vi "test_Remove Speciality Input Channels.vi"(8 "error in (no error)":errorcluster, 11 "TestCase in":refnum<class "FPGA Addon Adding Channel Items Unit Tests.lvclass">) -> (0 "error out":errorcluster, 3 "TestCase out":refnum<class "FPGA Addon Adding Channel Items Unit Tests.lvclass">)   [LabVIEW 2018, in "FPGA Addon Adding Channel Items Unit Tests.lvclass"]
uses:
  FPGA Addon Adding Channel Items Unit Tests.lvclass
  Addon/Addon Shared/Types/FG Action.ctl
  FPGA Addon Adding Channel Items Unit Tests.lvclass/FPGA Addon Adding Channel Items Unit Tests.ctl
  Addon/Addon Shared/SubVIs/Constants.vi
  <vilib>/NI Veristand/Custom Device Tools/Custom Device Utility Library/NI VeriStand - Search for Item by GUID.vi
  <vilib>/NI/NI VeriStand Advanced SysDef API/SysDef API/SysDef.Property.Get.vi
  <vilib>/NI/NI VeriStand Advanced SysDef API/_SubVIs/SysDef.Property.Get.Variant.vi
  <vilib>/NI/NI VeriStand Advanced SysDef API/SysDef API/SysDef.Property.Set.vi
  <vilib>/NI/NI VeriStand Advanced SysDef API/_SubVIs/SysDef.Property.Set.Variant.vi
  <vilib>/NI/NI VeriStand Advanced SysDef API/_SubVIs/SysDef.Search.GUIDs.vi
  <vilib>/addons/_JKI Toolkits/VI Tester/TestCase.llb/TestCase.lvclass
  Addon/Addon System Explorer/FPGA Addon System Explorer.lvlib
  Addon/Addon Shared/FPGA Addon Shared.lvlib
  <vilib>/NI Veristand/Custom Device Tools/Custom Device Utility Library/Custom Device Utility Library.lvlib
  <vilib>/NI/NI VeriStand Advanced SysDef API/SysDef API/Advanced System Definition.lvlib
  C:/Program Files (x86)/National Instruments/LabVIEW 2018/vi.lib/addons/_JKI Toolkits/VI Tester/TestCase.llb/TestCase.lvclass
panel:
  out "GUIDs":string[](array[string])
  in  "remove":bool
  in  "add":bool
  out "Names":string[](array[string])
  in  "Available Registers":i32[](listbox)
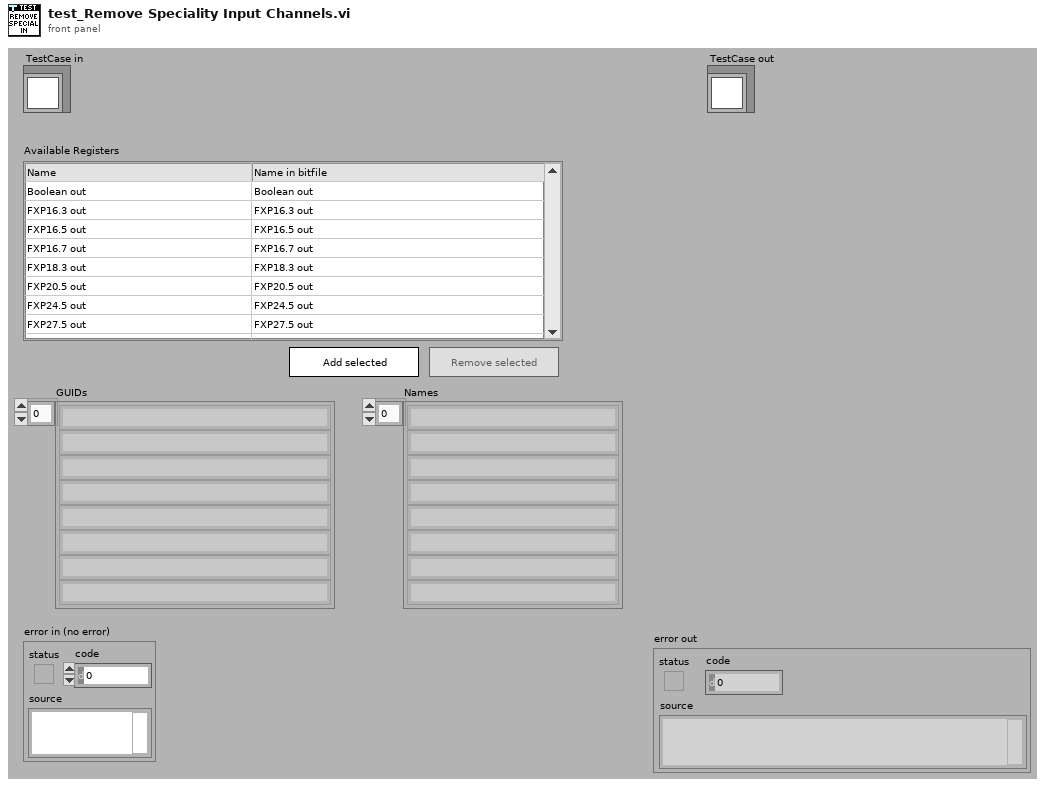
[diagram p1: front panel]
types:
  T1 = typedef "FPGA Addon Shared.lvlib/FG Action.ctl" = enum8{"GET", "SET"}
  T2 = typedef "Custom Device API.lvlib/Custom Device Item Ref.ctl" = u64
  T3 = typedef "FPGA Addon Shared.lvlib/Register Information.ctl" = cluster{"Name":string, "Data Type":T4, "Default Value":variant}
  T4 = typedef "FPGA Addon Shared.lvlib/Data Type.ctl" = enum8{"<Null>", "I8", "I16", "I32", "I64", "U8", "U16", "U32", "U64", "SGL", "Boolean", "Analog PWM In Settings", "Analog PWM In", "Digital PWM In Settings", "Digital PWM In", "Digital PWM Out", "Sine Out", "FXP+/-24.5", "FXP+/-16.5", "FXP+/-32.8", "FXP+/-64.32", "FXP+/-16.7", "FXP+/-20.5", "FXP+/-27.5", "FXP+/-32.16", "FXP+16.3", "FXP+18.3", "Digital Static In", "Digital Static Out", "Digital Static In Settings", "Digital WSS Out", "Quad Encoder Settings", "Quad Encoder In", "Group"}
  T5 = typedef "FPGA Addon System Explorer.lvlib/Listbox Cluster.ctl" = cluster{"add":refnum<vi>, "remove":refnum<vi>, "Listbox":refnum<vi>, "selected":i32[], "not present":i32[], "listbox text":string[][], "Section Ref":T2}
  T6 = typedef "Advanced System Definition.lvlib/TreeItem.Info.ctl" = cluster{"Name":string, "Description":string, "GUID":string, "Is Channel":bool, "Channel":T7, "Is Waveform":bool, "Waveform":T9}
  T7 = typedef "Custom Device API.lvlib/Custom Device Channel.ctl" = cluster{"Type":T8, "Units":string, "Default Value":dbl, "Faultable":bool, "Scalable":bool}
  T8 = typedef "Custom Device API.lvlib/Custom Device Channel Type.ctl" = enum16{"Input", "Output"}
  T9 = typedef "Custom Device API.lvlib/Custom Device Waveform.ctl" = cluster{"Data Type":T10, "Units":string}
  T10 = typedef "Custom Device API.lvlib/Custom Device Waveform DataType.ctl" = enum16{"Double", "Complex Double"}
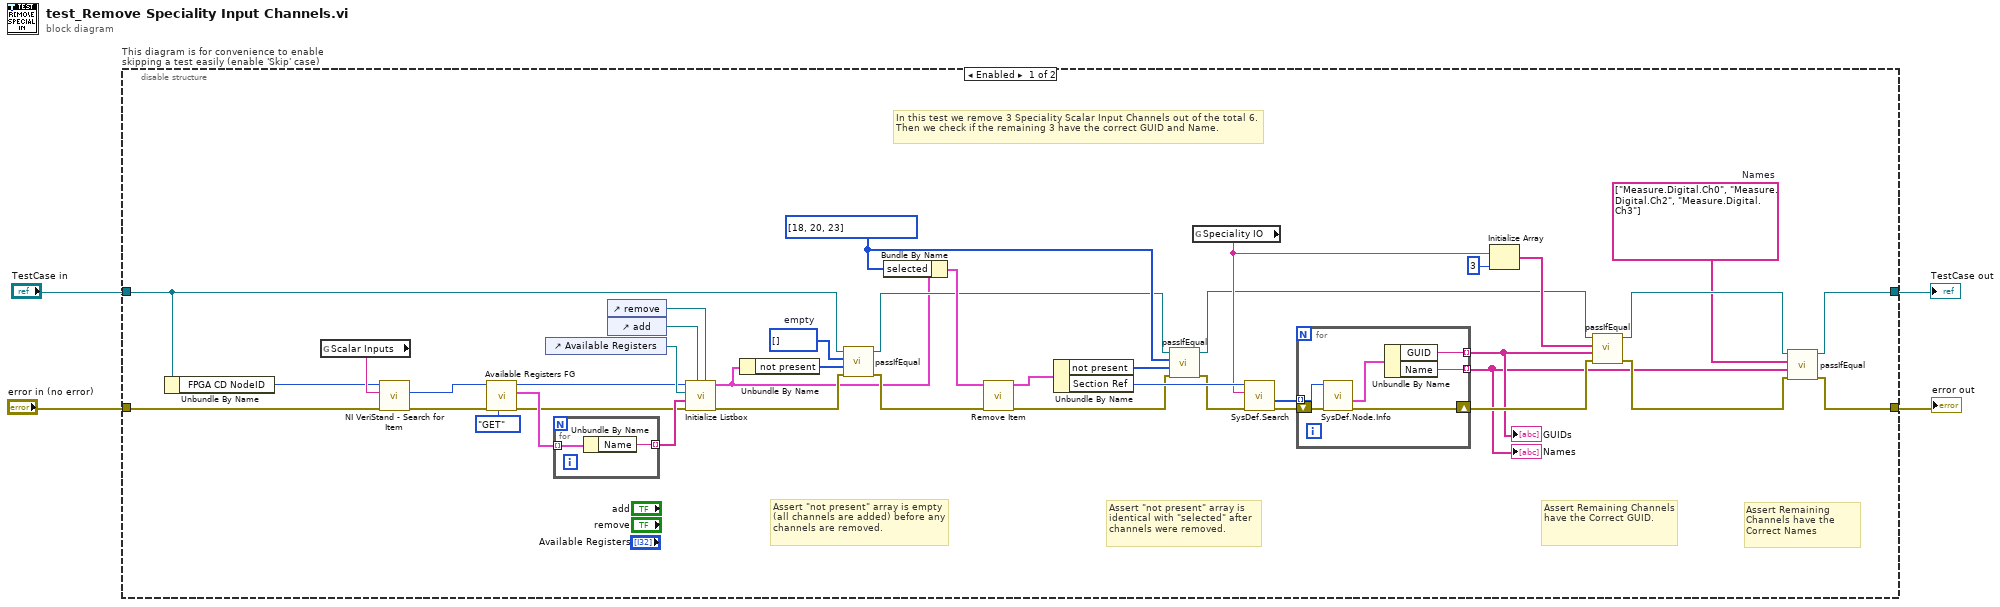
[diagram p0: block diagram]
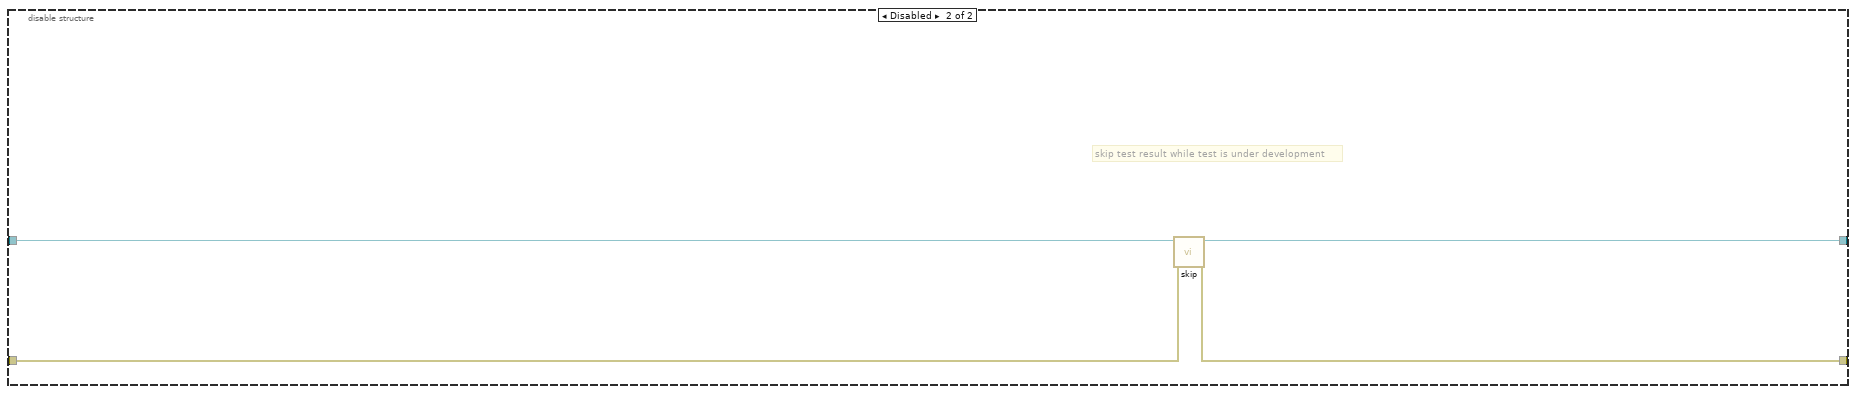
[diagram p2: hidden frame]
diagram:
  n1 = disable-structure "This diagram is for convenience to enable skipping a test easily (enable 'Skip' case)" shown="Enabled" {
    disable-tunnel: "TestCase in" -> [w9 w57]
    disable-tunnel: [w25 w55] -> w1
    disable-tunnel: [w24 w56] -> w3
    disable-tunnel: "error in (no error)" -> [w23 w54]
    frame Enabled {
      w10 = i32[] []  # empty
      w26 = string[] ["Measure.Digital.Ch0", "Measure.Digital.Ch2", "Measure.Digital.Ch3"]  # Names
      w12 = i32[] [18, 20, 23] ("selected")
      # "Assert \"not present\" array is empty (all channels are added) before any channels are removed."
      # "Assert \"not present\" array is identical with \"selected\" after channels were removed."
      # "In this test we remove 3 Speciality Scalar Input Channels out of the total 6. Then we check if the remaining 3 have the correct GUID and Name."
      # "Assert Remaining Channels have the Correct Names"
      # "Assert Remaining Channels have the Correct GUID."
      n2 = Unbundle By Name(w9) -> ("FPGA CD NodeID"=w22:u64)
      n3 = global read "Constants.vi" "Scalar Inputs"() -> (w41:string)
      n4 = call-poly <vilib>:"NI VeriStand - Search for Item.vi"("error in"=w23, "Item GUID"=w41, "Section Ref in"=w22) -> ("error out"=w40:errorcluster, "Item Ref"=w36:T2)  [unwired: 5 in, 2 out]
      n5 = call "Available Registers FG.vi"("Action"=FG_Action."GET", "error in (no error)"=w40, "Item Ref"=w36) -> ("error out"=w39:errorcluster, "Available Registers"=w43:T3[], "Item Ref out"=w38:T2)  [unwired: 6 in]
      n6 = control-ref of="Available Registers"() -> (w45:refnum<vi>)
      n7 = for {
        tunnel: w43 -> [w47] mode=indexing
        tunnel: [w46] -> w42 mode=indexing
        n8 = Unbundle By Name(w47) -> ("Name"=w46:string)
      }
      n9 = control-ref of="remove"() -> (w33:refnum<vi>)
      n10 = control-ref of="add"() -> (w34:refnum<vi>)
      n11 = call "Initialize Listbox.vi"("remove"=w33, "add"=w34, "error in (no error)"=w39, "Names"=w42, "Listbox"=w45, "Item Ref"=w38) -> ("error out"=w7:errorcluster, "Listbox Refs"=w5:T5)  [unwired: 4 in]
      n12 = Unbundle By Name(w5) -> ("not present"=w11:i32[])
      n13 = call-dynamic "passIfEqual.vi"("error in (no error)"=w7, "y"=w11, "x"=w10, "TestCase in"=w9) -> ("error out"=w6:errorcluster, "TestCase out"=w8:refnum<class "FPGA Addon Adding Channel Items Unit Tests.lvclass">)  [unwired: 6 in]
      n14 = Bundle By Name(cluster=w5, "selected"=w12) -> (w19:T5)
      n15 = call "Remove Item.vi"("error in (no error)"=w6, "Listbox Refs in"=w19) -> ("error out"=w16:errorcluster, "Listbox Refs out"=w18:T5)  [unwired: 8 in]
      n16 = Unbundle By Name(w18) -> ("not present"=w14:i32[], "Section Ref"=w35:T2)
      n17 = call-dynamic "passIfEqual.vi"("error in (no error)"=w16, "y"=w14, "x"=w12, "TestCase in"=w8) -> ("error out"=w15:errorcluster, "TestCase out"=w13:refnum<class "FPGA Addon Adding Channel Items Unit Tests.lvclass">)  [unwired: 6 in]
      n18 = global read "Constants.vi" "Speciality IO"() -> (w20:string)
      n19 = call-poly <vilib>:"SysDef.Search.vi"("error in (no error)"=w15, "GUID"=w20, "nodeID"=w35) -> ("error out"=w37:errorcluster, "Values Out"=w32:u64[])  [unwired: 5 in, 2 out]
      n20 = for {
        tunnel: w32 -> [w50] mode=indexing
        tunnel: [w48] -> w27 mode=indexing
        tunnel: [w49] -> w29 mode=indexing
        shift-right: [w52] -> w30
        shift-left: w37 -> [w53]
        n21 = call <vilib>:"SysDef.Node.Info.vi"("error in (no error)"=w53, "nodeID"=w50) -> ("error out"=w52:errorcluster, "Item Info"=w51:T6)  [unwired: 6 in, 2 out]
        n22 = Unbundle By Name(w51) -> ("GUID"=w49:string, "Name"=w48:string)
      }
      "Names" <- w27
      "GUIDs" <- w29
      n23 = Initialize Array(w20, 3 ("dimension size")) -> (w21:string[])
      n24 = call-dynamic "passIfEqual.vi"("error in (no error)"=w30, "y"=w29, "x"=w21, "TestCase in"=w13) -> ("error out"=w31:errorcluster, "TestCase out"=w28:refnum<class "FPGA Addon Adding Channel Items Unit Tests.lvclass">)  [unwired: 6 in]
      n25 = call-dynamic "passIfEqual.vi"("error in (no error)"=w31, "y"=w27, "x"=w26, "TestCase in"=w28) -> ("error out"=w24:errorcluster, "TestCase out"=w25:refnum<class "FPGA Addon Adding Channel Items Unit Tests.lvclass">)  [unwired: 6 in]
    }
    frame Disabled {
      # "skip test result while test is under development"
      n26 = call <vilib>:"skip.vi"("error in (no error)"=w54, "TestCase in"=w57) -> ("error out"=w56:errorcluster, "TestCase out"=w55:refnum<class "FPGA Addon Adding Channel Items Unit Tests.lvclass">)  [unwired: 8 in]
    }
  }
  "error out" <- w3
  "TestCase out" <- w1
